vi "Source_Q_wrong.vi"(2 "Ch Names":string[](array[string]), 3 "Values":dbl[](array[numeric]) format="%.2f") -> (0 "Gas Error?":bool)   [LabVIEW 2014]
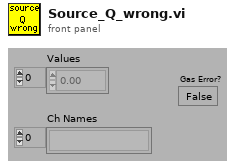
[diagram p1: front panel]
types:
  T1 = enum16{"Append to Global", "Read Global then Clear"}
  T2 = typedef "Ch_description_ADAM.ctl" = cluster{"Ch Name":string, "Type":T3, "Function":T4, "Ch State":T5, "Calibration type":T6, "A":dbl, "B":dbl, "C":dbl, "D":dbl, "Comments":string, "Address":T7, "String":string, "Duty":u16}
  T3 = typedef "Module_type_ADAM.ctl" = string
  T4 = typedef "Function_ADAM.ctl" = enum16{"Analogue Input", "Digital Input", "Event counter", "Event rate", "Analogue Output", "Digital Output", "Relay Output"}
  T5 = typedef "Channel_State.ctl" = enum16{"On", "Off", "Always On", "Always Off"}
  T6 = typedef "Calib_type_ADAM.ctl" = enum16{"Raw", "Bx + A", "Cx^2 + Bx + A", "Dx^3 + Cx^2 + Bx + A", "In Band", "Hi-Tec Q", "Hi-Tec M_dot", "Text"}
  T7 = typedef "Address.ctl" = cluster{"Main":i32, "Ch.":i32, "Sub":i32, "Port Name":string}
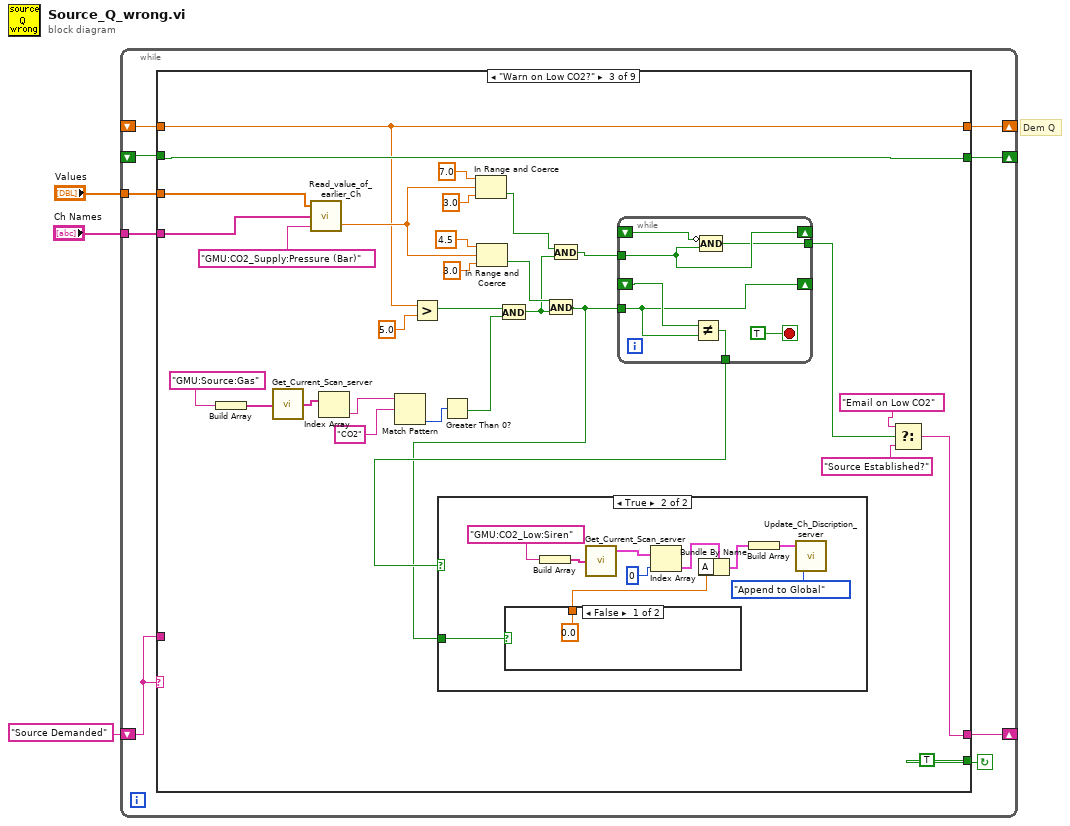
[diagram p0: block diagram]
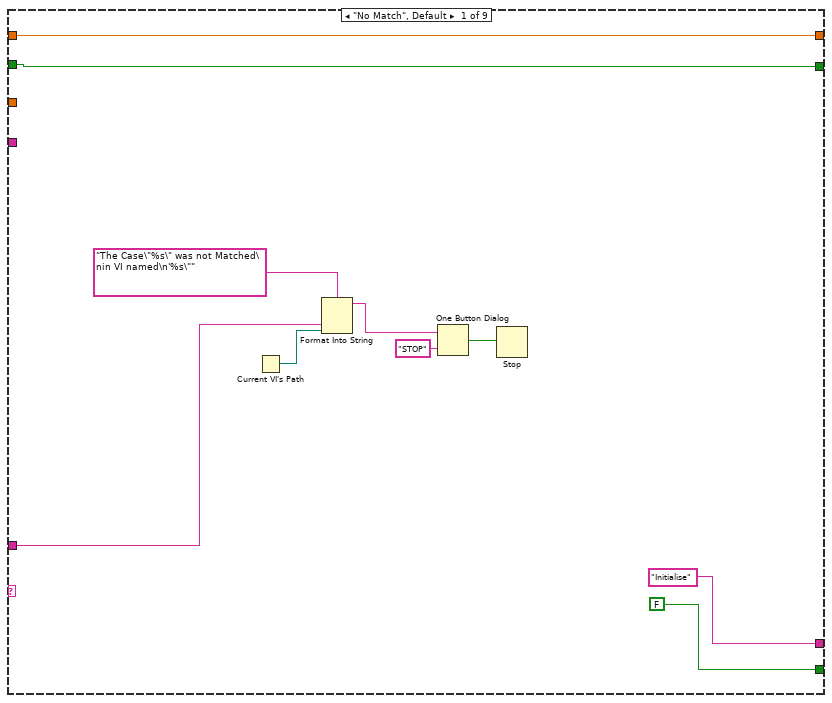
[diagram p2: hidden frame]
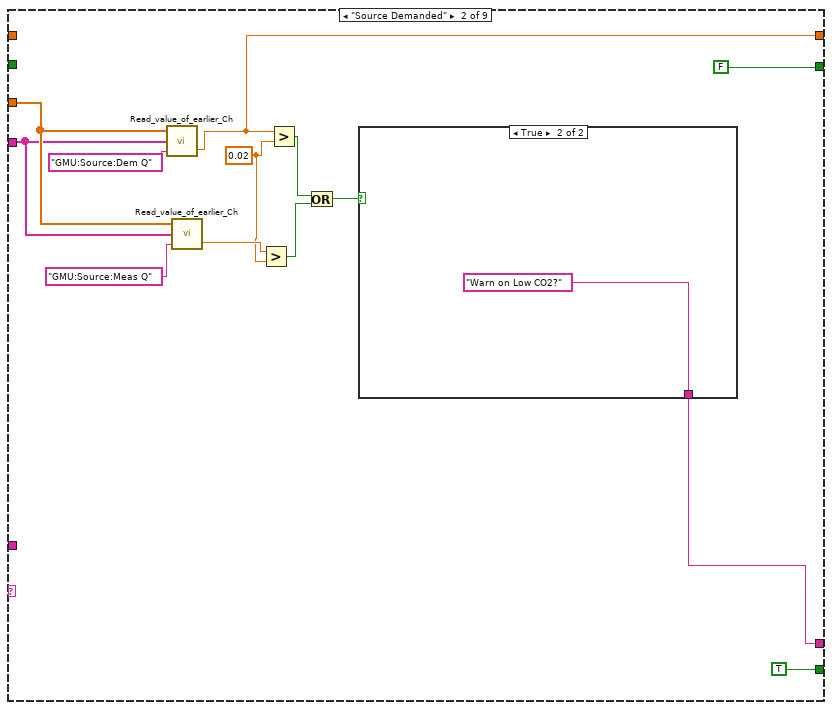
[diagram p3: hidden frame]
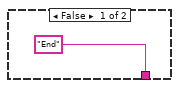
[diagram p4: hidden frame]
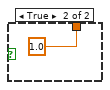
[diagram p6: hidden frame]
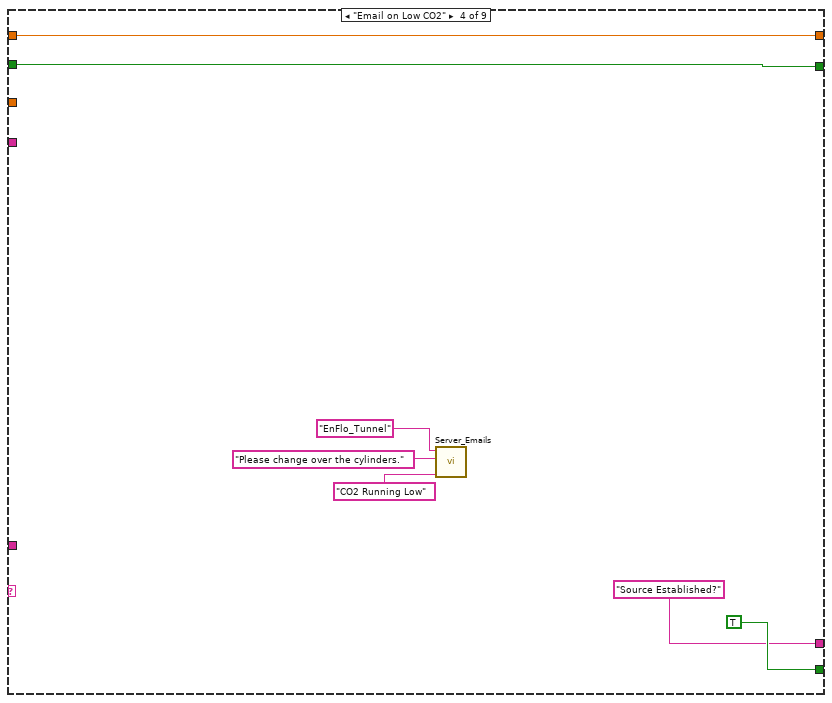
[diagram p7: hidden frame]
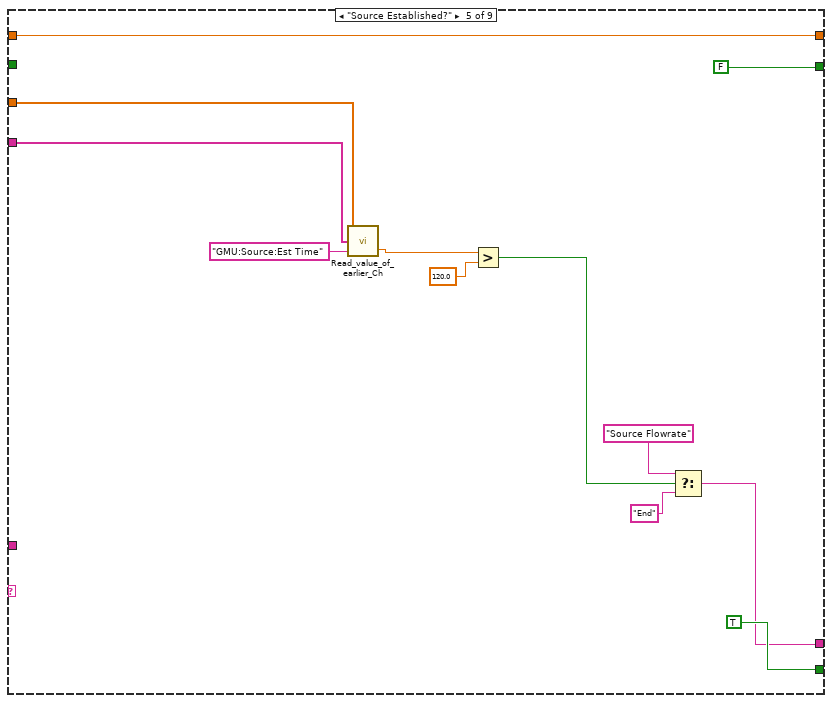
[diagram p8: hidden frame]
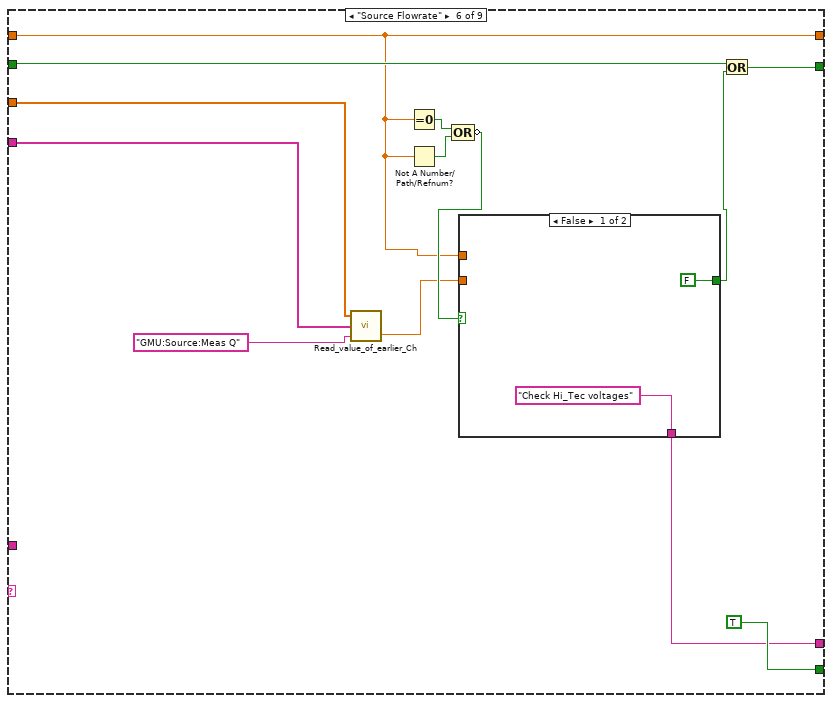
[diagram p9: hidden frame]
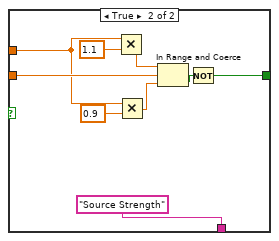
[diagram p10: hidden frame]
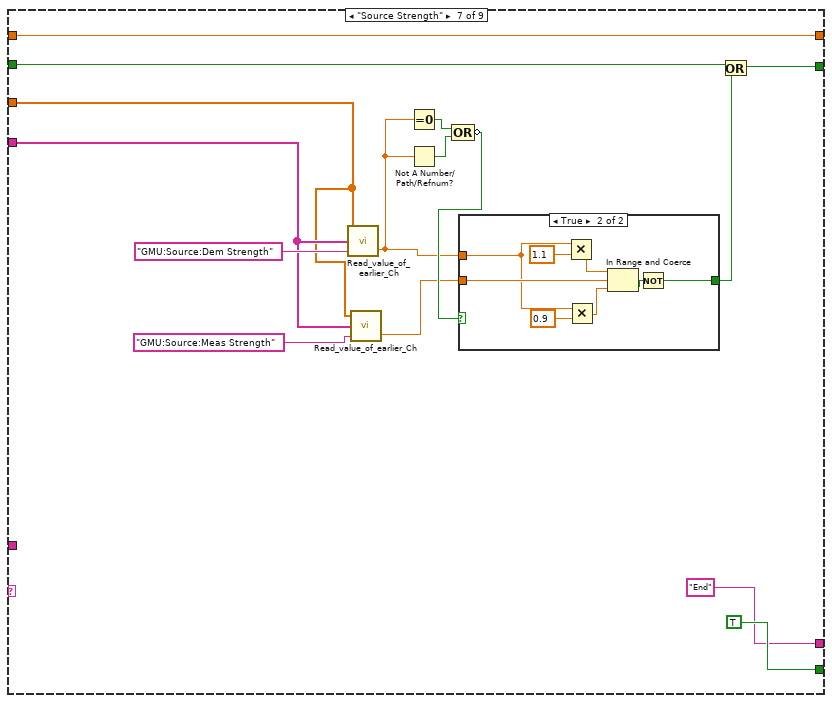
[diagram p11: hidden frame]
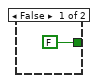
[diagram p12: hidden frame]
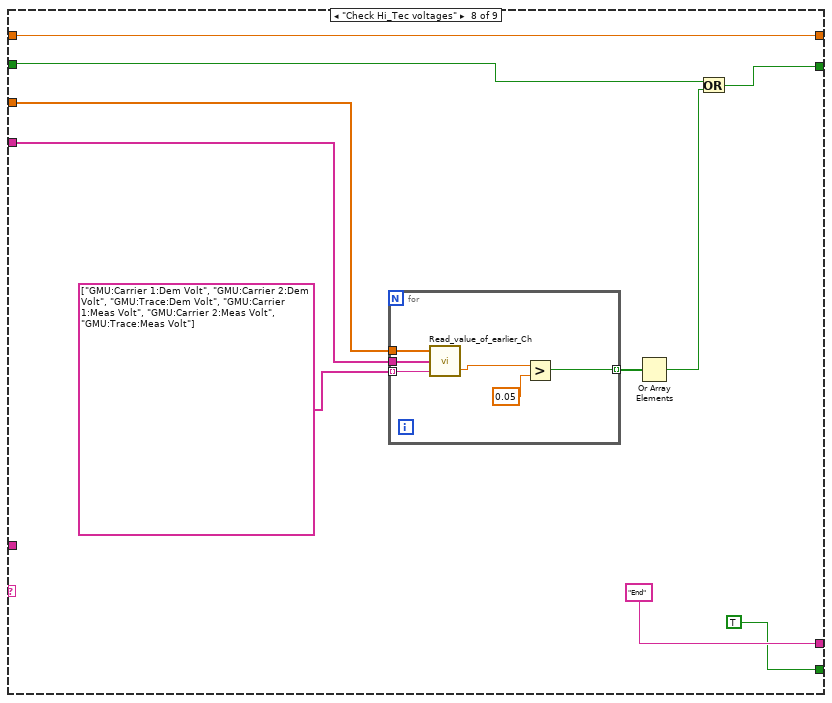
[diagram p13: hidden frame]
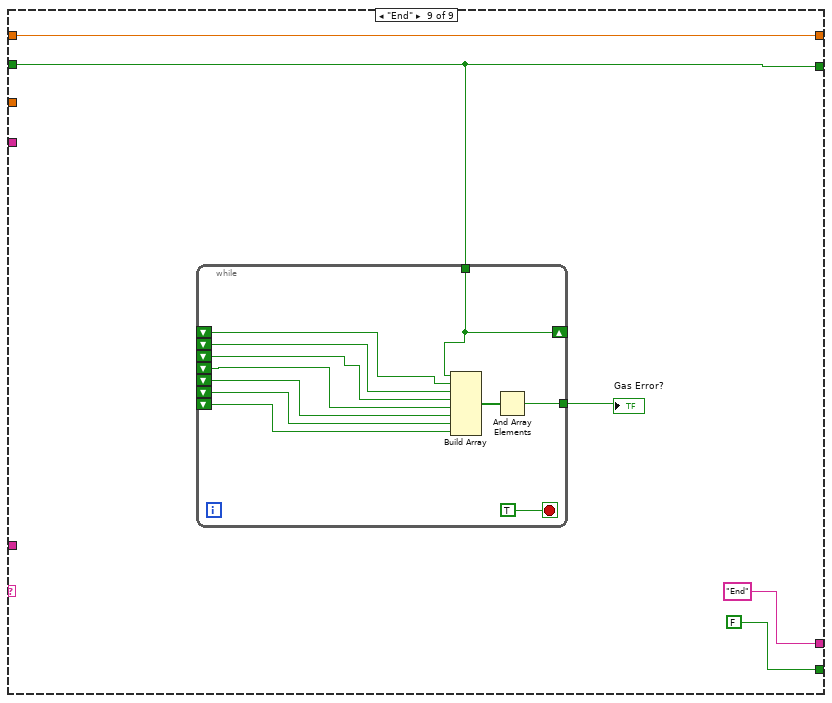
[diagram p14: hidden frame]
diagram:
  # "Dem Q"
  n1 = while {
    shift-left: "Source Demanded" -> [w10]
    shift-right: [w11] -> _
    tunnel: "Ch Names" -> [w9]
    tunnel: "Values" -> [w8]
    shift-right: [w7] -> _
    shift-left: _ -> [w6]
    shift-right: [w5] -> _
    shift-left: _ -> [w4]
    stop <- w12 continue-if-true
    n2 = case shown="\"Warn on Low CO2?\"" w10 {
      tunnel: [FALSE TRUE TRUE TRUE TRUE TRUE TRUE TRUE FALSE] -> w12
      tunnel: ["Initialise" w24 w41 "Source Established?" w96 w107 "End" ("f") "End" "End" ("f")] -> w11
      tunnel: w10 -> [w17 _ _ _ _ _ _ _ _]
      tunnel: w9 -> [_ w30 w62 _ w104 w117 w133 w161 _]
      tunnel: w8 -> [_ w31 w61 _ w103 w118 w132 w159 _]
      tunnel: [w14 FALSE w39 w92 FALSE w110 w134 w155 w172] -> w7
      tunnel: w6 -> [w14 _ w39 w92 _ w108 w135 w156 w172]
      tunnel: [w13 w32 w38 w87 w94 w106 w130 w154 w170] -> w5
      tunnel: w4 -> [w13 _ w38 w87 w94 w106 w130 w154 w170]
      frame "No Match", Default {
        n3 = Current VI's Path() -> (path=w16:path)
        n4 = Format Into String(format string="The Case\"%s\" was not Matched\nin VI named\n'%s\"" ("Format String"), w17, w16) -> (resulting string=w20:string)  [unwired: 2 in, 1 out]
        n5 = One Button Dialog(message=w20, button name ("OK")="STOP") -> (true=w18:bool)
        n6 = Stop(stop? (T)=w18) -> ()
      }
      frame "Source Demanded" {
        w27 = 0.02 ("y")
        n7 = call "Read_value_of_earlier_Ch.vi"("Desired Ch to Read"="GMU:Source:Dem Q", "Ch names"=w30, "Present scan array"=w31) -> ("Value"=w32:dbl)  [unwired: 1 in, 1 out]
        n8 = call "Read_value_of_earlier_Ch.vi"("Desired Ch to Read"="GMU:Source:Meas Q", "Ch names"=w30, "Present scan array"=w31) -> ("Value"=w28:dbl)  [unwired: 1 in, 1 out]
        n9 = Greater?(x=w28, y=w27) -> (0:w23:bool)
        n10 = Greater?(x=w32, y=w27) -> (0:w26:bool)
        n11 = Or(x=w26, y=w23) -> (x .or. y?=w25:bool)
        n12 = case shown="True" w25 {
          tunnel: ["End" "Warn on Low CO2?"] -> w24
          frame False {
          }
          frame True {
          }
        }
      }
      frame "Warn on Low CO2?" {
        n13 = Build Array("GMU:Source:Gas") -> (w58:string[])
        n14 = call "Get_Current_Scan_server.vi"("Desired Channels"=w58) -> ("String values"=w57:string[])  [unwired: 2 out]
        n15 = call "Read_value_of_earlier_Ch.vi"("Desired Ch to Read"="GMU:CO2_Supply:Pressure (Bar)", "Ch names"=w62, "Present scan array"=w61) -> ("Value"=w51:dbl)  [unwired: 1 in, 1 out]
        n16 = Index Array(array=w57) -> (element=w56:string)  [unwired: 1 in]
        n17 = Match Pattern(string=w56, regular expression="CO2") -> (offset past match=w54:i32)  [unwired: 1 in, 3 out]
        n18 = Greater?(x=w38, y=5.0) -> (0:w50:bool)
        n19 = Greater Than 0?(x=w54) -> (x > 0?=w49:bool)
        n20 = In Range and Coerce(upper limit=7.0, x=w51, lower limit=3.0) -> (In Range?=w48:bool)  [unwired: 1 out]
        n21 = In Range and Coerce(upper limit=4.5, x=w51, lower limit=3.0) -> (In Range?=w47:bool)  [unwired: 1 out]
        n22 = And(x=w50, y=w49) -> (x .and. y?=w45:bool)
        n23 = And(x=w47, y=w45) -> (x .and. y?=w46:bool)
        n24 = And(x=w48, y=w45) -> (x .and. y?=w44:bool)
        n25 = while {
          shift-right: [w84] -> _
          shift-left: _ -> [w85]
          tunnel: w46 -> [w84]
          tunnel: [w83] -> w60
          shift-right: [w82] -> _
          shift-left: _ -> [w81]
          tunnel: w44 -> [w82]
          tunnel: [w80] -> w43
          stop <- TRUE stop-if-true
          n26 = Not Equal?(x=w85, y=w84) -> (x != y?=w83:bool)
          n27 = Compound Arithmetic op=AND(invert w81, w82) -> (w80:bool)
        }
        n28 = case shown="True" w60 {
          tunnel: w46 -> [_ w76]
          frame False {
          }
          frame True {
            n29 = case shown="False" w76 {
              tunnel: [0.0 ("A") 1.0 ("A")] -> w71
              frame False {
              }
              frame True {
              }
            }
            n30 = Build Array("GMU:CO2_Low:Siren") -> (w75:string[])
            n31 = call "Get_Current_Scan_server.vi"("Desired Channels"=w75) -> ("Ch Description Array"=w74:T2[])  [unwired: 2 out]
            n32 = Index Array(array=w74, index=0) -> (element=w72:T2)
            n33 = Bundle By Name(cluster=w72, "A"=w71) -> (w69:T2)
            n34 = Build Array(w69) -> (w68:T2[])
            n35 = call "Update_Ch_Discription_server.vi"("Mode"=T1."Append to Global", "Channels to update In"=w68) -> ()  [unwired: 1 in, 1 out]
          }
        }
        n36 = Select(t="Email on Low CO2", s=w43, f="Source Established?") -> (s? t:f=w41:string)
      }
      frame "Email on Low CO2" {
        n37 = call "Server_Emails.vi"("Client Name Contains"="EnFlo_Tunnel", "Message"="Please change over the cylinders.", "Subject"="CO2 Running Low") -> ()  [unwired: 2 in, 3 out]
      }
      frame "Source Established?" {
        n38 = call "Read_value_of_earlier_Ch.vi"("Desired Ch to Read"="GMU:Source:Est Time", "Ch names"=w104, "Present scan array"=w103) -> ("Value"=w101:dbl)  [unwired: 1 in, 1 out]
        n39 = Greater?(x=w101, y=120.0) -> (0:w98:bool)
        n40 = Select(t="Source Flowrate", s=w98, f="End") -> (s? t:f=w96:string)
      }
      frame "Source Flowrate" {
        n41 = call "Read_value_of_earlier_Ch.vi"("Desired Ch to Read"="GMU:Source:Meas Q", "Ch names"=w117, "Present scan array"=w118) -> ("Value"=w112:dbl)  [unwired: 1 in, 1 out]
        n42 = Equal To 0?(x=w106) -> (x = 0?=w115:bool)
        n43 = Not A Number/Path/Refnum?(number/path/refnum=w106) -> (NaN/Path/Refnum?=w114:bool)
        n44 = Compound Arithmetic op=OR(w115, w114) -> (invert w113:bool)
        n45 = case shown="False" w113 {
          tunnel: w112 -> [_ w125]
          tunnel: w106 -> [_ w124]
          tunnel: [FALSE w122] -> w109
          tunnel: ["Check Hi_Tec voltages" "Source Strength"] -> w107
          frame False {
          }
          frame True {
            n46 = Multiply(x=w124, y=1.1) -> (x*y=w129:dbl)
            n47 = Multiply(x=w124, y=0.9) -> (x*y=w128:dbl)
            n48 = In Range and Coerce(upper limit=w129, x=w125, lower limit=w128) -> (In Range?=w123:bool)  [unwired: 1 out]
            n49 = Not(x=w123) -> (.not. x?=w122:bool)
          }
        }
        n50 = Or(x=w108, y=w109) -> (x .or. y?=w110:bool)
      }
      frame "Source Strength" {
        n51 = call "Read_value_of_earlier_Ch.vi"("Desired Ch to Read"="GMU:Source:Dem Strength", "Ch names"=w133, "Present scan array"=w132) -> ("Value"=w139:dbl)  [unwired: 1 in, 1 out]
        n52 = call "Read_value_of_earlier_Ch.vi"("Desired Ch to Read"="GMU:Source:Meas Strength", "Ch names"=w133, "Present scan array"=w132) -> ("Value"=w138:dbl)  [unwired: 1 in, 1 out]
        n53 = Equal To 0?(x=w139) -> (x = 0?=w142:bool)
        n54 = Not A Number/Path/Refnum?(number/path/refnum=w139) -> (NaN/Path/Refnum?=w141:bool)
        n55 = Compound Arithmetic op=OR(w142, w141) -> (invert w140:bool)
        n56 = case shown="True" w140 {
          tunnel: w138 -> [_ w149]
          tunnel: w139 -> [_ w148]
          tunnel: [FALSE w146] -> w136
          frame False {
          }
          frame True {
            n57 = Multiply(x=w148, y=1.1) -> (x*y=w153:dbl)
            n58 = Multiply(x=w148, y=0.9) -> (x*y=w152:dbl)
            n59 = In Range and Coerce(upper limit=w153, x=w149, lower limit=w152) -> (In Range?=w147:bool)  [unwired: 1 out]
            n60 = Not(x=w147) -> (.not. x?=w146:bool)
          }
        }
        n61 = Or(x=w135, y=w136) -> (x .or. y?=w134:bool)
      }
      frame "Check Hi_Tec voltages" {
        n62 = for {
          tunnel: w159 -> [w169]
          tunnel: w161 -> [w168]
          tunnel: string[] ["GMU:Carrier 1:Dem Volt", "GMU:Carrier 2:Dem Volt", "GMU:Trace:Dem Volt", "GMU:Carrier 1:Meas Volt", "GMU:Carrier 2:Meas Volt", "GMU:Trace:Meas Volt"] ("appended array") -> [w167] mode=indexing
          tunnel: [w164] -> w158 mode=indexing
          n63 = call "Read_value_of_earlier_Ch.vi"("Desired Ch to Read"=w167, "Ch names"=w168, "Present scan array"=w169) -> ("Value"=w165:dbl)  [unwired: 1 in, 1 out]
          n64 = Greater?(x=w165, y=0.05) -> (0:w164:bool)
        }
        n65 = Or Array Elements(Boolean array=w158) -> (logical OR=w157:bool)
        n66 = Or(x=w156, y=w157) -> (x .or. y?=w155:bool)
      }
      frame "End" {
        n67 = while {
          shift-right: [w184] -> _
          shift-left: _ -> [w183]
          shift-left: _ -> [w182]
          shift-left: _ -> [w181]
          shift-left: _ -> [w180]
          shift-left: _ -> [w179]
          shift-left: _ -> [w178]
          shift-left: _ -> [w177]
          tunnel: w172 -> [w184]
          tunnel: [w175] -> w174
          stop <- TRUE stop-if-true
          n68 = Build Array(w184, w183, w182, w181, w180, w179, w178, w177) -> (w176:bool[])
          n69 = And Array Elements(Boolean array=w176) -> (logical AND=w175:bool)
        }
        "Gas Error?" <- w174
      }
    }
  }
